vi "실적확인.vi"() -> ()   [LabVIEW 2020]
uses:
  <vilib>/addons/database/NI_Database_API.lvlib
panel:
  in  "정지":bool
  out "Elapsed Time (s)":dbl caption="경과 시간(초)"
  out "QUERY":string
  out "숫자형 2":i32
  out "숫자형":i32
  in  "링":u16(ring) items=["2018"=2018, "2019"=2019, "2020"=2020, "2021"=2021]
  out "Data":string[][](array[string])
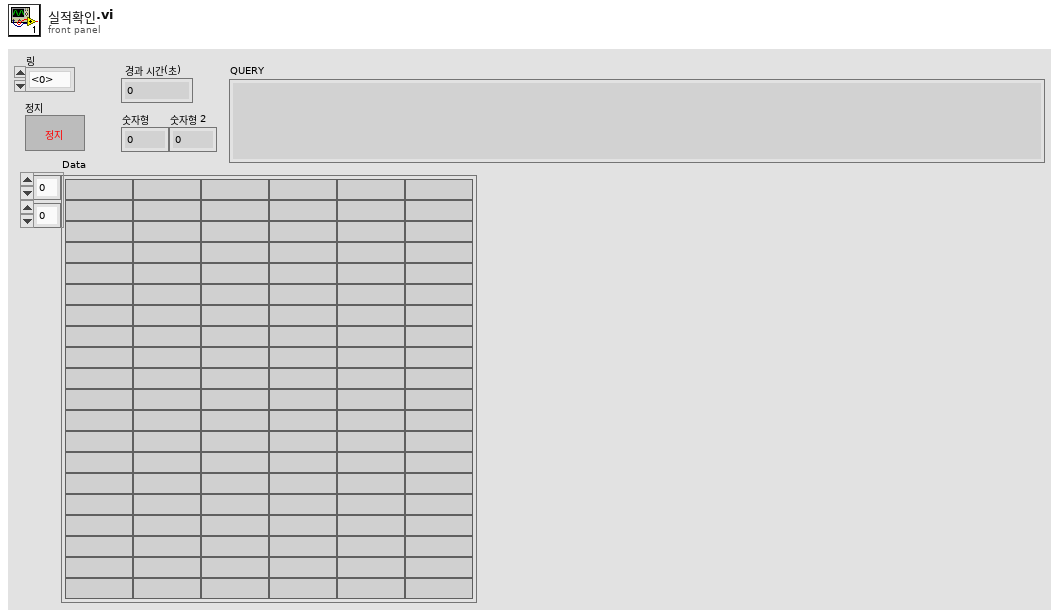
[diagram p1: front panel]
types:
  T1 = typedef "NI_Database_API.lvlib/Conn ObjectReference.ctl" = refnum<k1>
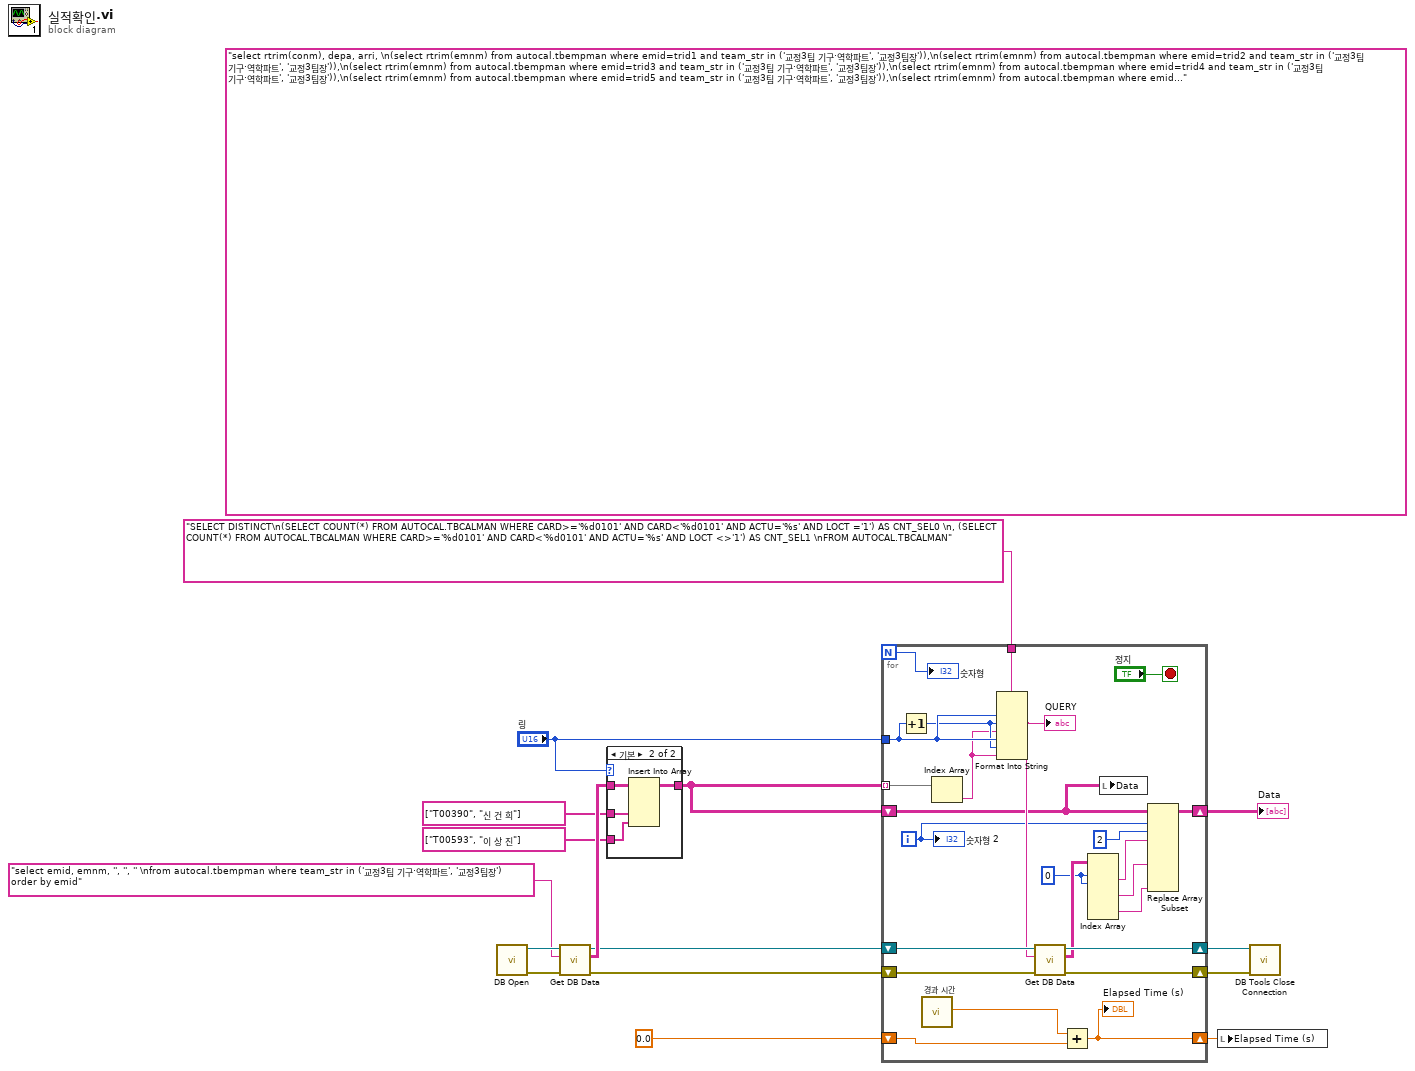
[diagram p0: block diagram]
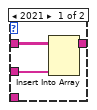
[diagram p2: hidden frame]
diagram:
  (unwired) "select rtrim(conm), depa, arri, \n(select rtrim(emnm) from autocal.tbempman where emid=trid1 and team_str in ('교정3팀 기구·역학파트', '교정3팀장')),\n(select rtrim(emnm) from autocal.tbempman where emid=trid2 and team_str in ('교정3팀 기구·역학파트', '교정3팀장')),\n(select rtrim(emnm) from autocal.tbempman where emid=trid3 and team_str in ('교정3팀 기구·역학파트', '교정3팀장')),\n(select rtrim(emnm) from autocal.tbempman where emid=trid4 and team_str in ('교정3팀 기구·역학파트', '교정3팀장')),\n(select rtrim(emnm) from autocal.tbempman where emid=trid5 and team_str in ('교정3팀 기구·역학파트', '교정3팀장')),\n(select rtrim(emnm) from autocal.tbempman where emid=trid6 and team_str in ('교정3팀 기구·역학파트', '교정3팀장')),\n((select count(emnm) from autocal.tbempman where emid=trid1 and team_str in ('교정3팀 기구·역학파트', '교정3팀장'))\n+(select count(emnm) from autocal.tbempman where emid=trid2 and team_str in ('교정3팀 기구·역학파트', '교정3팀장'))\n+(select count(emnm) from autocal.tbempman where emid=trid3 and team_str in ('교정3팀 기구·역학파트', '교정3팀장'))\n+(select count(emnm) from autocal.tbempman where emid=trid4 and team_str in ('교정3팀 기구·역학파트', '교정3팀장'))\n+(select count(emnm) from autocal.tbempman where emid=trid5 and team_str in ('교정3팀 기구·역학파트', '교정3팀장'))\n+(select count(emnm) from autocal.tbempman where emid=trid6 and team_str in ('교정3팀 기구·역학파트', '교정3팀장'))),\nTO_DATE(arri,'yyyymmdd')-TO_DATE(depa,'yyyymmdd')+1,\n((select count(isid) from autocal.tbcalman where actu=(select emid from autocal.tbempman where emid=trid1 and team_str in ('교정3팀 기구·역학파트', '교정3팀장')) and card>=depa and card<=arri and ccom=coid)\n+(select count(isid) from autocal.tbcalman where actu=(select emid from autocal.tbempman where emid=trid2 and team_str in ('교정3팀 기구·역학파트', '교정3팀장')) and card>=depa and card<=arri and ccom=coid)\n+(select count(isid) from autocal.tbcalman where actu=(select emid from autocal.tbempman where emid=trid3 and team_str in ('교정3팀 기구·역학파트', '교정3팀장')) and card>=depa and card<=arri and ccom=coid)\n+(select count(isid) from autocal.tbcalman where actu=(select emid from autocal.tbempman where emid=trid4 and team_str in ('교정3팀 기구·역학파트', '교정3팀장')) and card>=depa and card<=arri and ccom=coid)\n+(select count(isid) from autocal.tbcalman where actu=(select emid from autocal.tbempman where emid=trid5 and team_str in ('교정3팀 기구·역학파트', '교정3팀장')) and card>=depa and card<=arri and ccom=coid)\n+(select count(isid) from autocal.tbcalman where actu=(select emid from autocal.tbempman where emid=trid6 and team_str in ('교정3팀 기구·역학파트', '교정3팀장')) and card>=depa and card<=arri and ccom=coid))\nfrom autocal.tbtripsh a, autocal.tbsupman b\nwhere\n(trid1 in (select emid from autocal.tbempman where team_str in ('교정3팀 기구·역학파트', '교정3팀장'))\nor trid2 in (select emid from autocal.tbempman where team_str in ('교정3팀 기구·역학파트', '교정3팀장'))\nor trid3 in (select emid from autocal.tbempman where team_str in ('교정3팀 기구·역학파트', '교정3팀장'))\nor trid4 in (select emid from autocal.tbempman where team_str in ('교정3팀 기구·역학파트', '교정3팀장'))\nor trid5 in (select emid from autocal.tbempman where team_str in ('교정3팀 기구·역학파트', '교정3팀장'))\nor trid6 in (select emid from autocal.tbempman where team_str in ('교정3팀 기구·역학파트', '교정3팀장')))\n\nand cust in (select coid from autocal.TBSUPMAN where ind_type ='C')\nand cust=coid\nand depa>='20201101' and depa<'20211101'\nand a.stat in ('출완  ', '접완  ')\n"
  n1 = call "DB Open.vi"() -> ("에러 출력"=w16:errorcluster, "참조 번호 출력"=w15:T1)  [unwired: 10 in]
  n2 = call "Get DB Data.vi"("error in (no error)"=w16, "SQL query"="select emid, emnm, '', '', '' \nfrom autocal.tbempman where team_str in ('교정3팀 기구·역학파트', '교정3팀장') order by emid", "connection reference"=w15) -> ("error out"=w8:errorcluster, "Data"=w13:string[][], "connection reference"=w10:T1)  [unwired: 4 in, 2 out]
  n3 = case shown="기본" "링" {
    tunnel: [w19 w23] -> w5
    tunnel: w13 -> [w18 w22]
    tunnel: string[] ["T00390", "신 건 희"] ("새 원소/부분배열") -> [w17 w21]
    tunnel: string[] ["T00593", "이 상 진"] ("새 원소/부분배열") -> [_ w20]
    frame 2021 {
      n4 = Insert Into Array(array=w18, new element=w17) -> (w19:string[][])  [unwired: 2 in]
    }
    frame Default {
      n5 = Insert Into Array(array=w22, new element #1=w21, new element #2=w20) -> (w23:string[][])  [unwired: 2 in]
    }
  }
  n6 = for {
    N -> [w41]
    shift-right: [w46] -> w9
    shift-left: w10 -> [w47]
    shift-right: [w44] -> w7
    shift-left: w8 -> [w45]
    tunnel: w5 -> [w36] mode=indexing
    tunnel: "SELECT DISTINCT\n(SELECT COUNT(*) FROM AUTOCAL.TBCALMAN WHERE CARD>='%d0101' AND CARD<'%d0101' AND ACTU='%s' AND LOCT ='1') AS CNT_SEL0 \n, (SELECT COUNT(*) FROM AUTOCAL.TBCALMAN WHERE CARD>='%d0101' AND CARD<'%d0101' AND ACTU='%s' AND LOCT <>'1') AS CNT_SEL1 \nFROM AUTOCAL.TBCALMAN" -> [w43]
    shift-right: [w37] -> w4
    shift-left: w5 -> [w35]
    tunnel: "링" -> [w29]
    shift-right: [w30] -> w1
    shift-left: 0.0 ("Elapsed Time (s)") -> [w32]
    i -> [w38]
    stop <- "정지" stop-if-true
    w39 = 0 ("인덱스 (행)")
    n7 = Increment(x=w29) -> (x+1=w28:u16)
    n8 = call "경과 시간"() -> ("Elapsed Time (s)"=w31:dbl)  [unwired: 12 in, 7 out]
    n9 = Index Array(array=w36) -> (element=w27:string)  [unwired: 1 in]
    n10 = Format Into String(format string=w43, w29, w28, w27, w29, w28, w27) -> (resulting string=w42:string)  [unwired: 2 in, 1 out]
    "QUERY" <- w42
    n11 = call "Get DB Data.vi"("error in (no error)"=w45, "SQL query"=w42, "connection reference"=w47) -> ("error out"=w44:errorcluster, "Data"=w40:string[][], "connection reference"=w46:T1)  [unwired: 4 in, 2 out]
    n12 = Add(x=w31, y=w32) -> (x+y=w30:dbl)
    "Elapsed Time (s)" <- w30
    n13 = Index Array(array=w40, index (row) #1=w39, index (col) #1=w39) -> (element #1=w33:string, element #2=w26:string, element #3=w25:string)  [unwired: 4 in]
    n14 = local write "Data"(w35) -> ()
    n15 = Replace Array Subset(array=w35, new element #1=w33, index (row) #1=w38, index (col) #1=2 ("비활성화된 인덱스 (열)"), new element #2=w26, new element #3=w25) -> (w37:string[][])  [unwired: 4 in]
    "숫자형" <- w41
    "숫자형 2" <- w38
  }
  "Data" <- w4
  n16 = local write "Elapsed Time (s)"(w1) -> ()
  n17 = call <vilib>:"DB Tools Close Connection.vi"("error in (no error)"=w7, "connection reference"=w9) -> ()  [unwired: 5 in, 1 out]
